vi "Test Publisher.vi"() -> ()   [LabVIEW 2021]
uses:
  CIFChannels/Typedef/Direction.ctl
  CIF_NIChn_FIFO_DAQ.lvclass
  ChannelCommon/typedef/TimeStamps.ctl
  ChannelCommon/typedef/Datatype Waveform.ctl
  <vilib>/CIF Foundation/CIF Utilities/DataTypes/Flatten U64.vi
  CIFChannels/CIFChannels.lvclass
  ChannelCommon/ChannelCommon.lvlib
panel:
  in  "stop":bool
  out "timed out?":bool
  out "error out":errorcluster
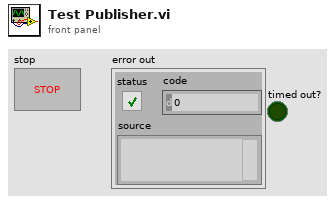
[diagram p1: front panel]
types:
  T1 = typedef "CIFChannels.lvclass/Direction.ctl" = enum16{"Publisher", "Subscriber"}
  T2 = typedef "ChannelCommon.lvlib/Datatype Waveform.ctl" = cluster{"measurement":dbl[], "dT":dbl, "Timestamp":i64, "Read Lock":bool}
  T3 = typedef "ChannelCommon.lvlib/TimeStamps.ctl" = cluster{"ClockID":u8, "T0":i64, "T_Out":i64}
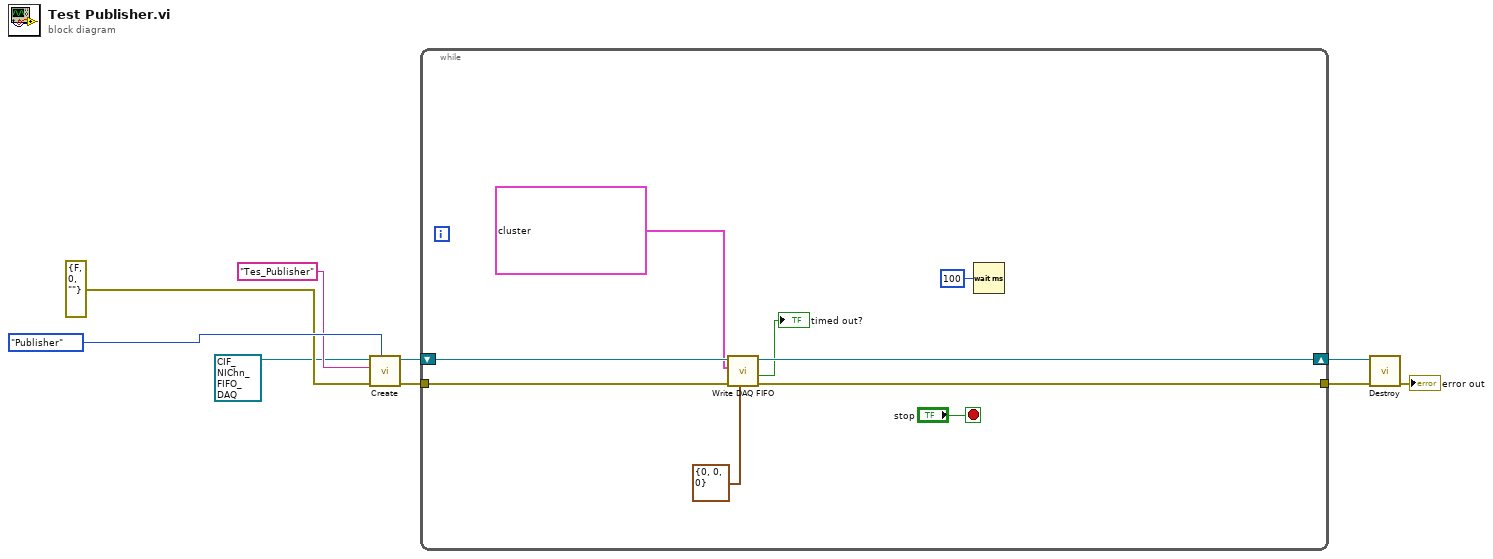
[diagram p0: block diagram]
diagram:
  n1 = call-dynamic "Create.vi"("Direction"=Direction."Publisher", "error in (no error)"=errorcluster {"status"=FALSE, "code"=0, "source"=""} ("error out"), "Name"="Tes_Publisher", "CIFFIFO in"=refnum<class "CIF_NIChn_FIFO_DAQ.lvclass"> refnum ("CIF_NIChn_FIFO_DAQ.lvclass")) -> ("error out"=w5:errorcluster, "CIFFIFO out"=w6:refnum<class "CIF_NIChn_FIFO_DAQ.lvclass">)  [unwired: 6 in]
  n2 = while {
    shift-right: [w15] -> w4
    shift-left: w6 -> [w17]
    tunnel: w5 -> [w16]
    tunnel: [w14] -> w3
    stop <- "stop" stop-if-true
    n3 = call-dynamic "Write DAQ FIFO.vi"("FIFO Timestamps"=T3 {"ClockID"=0, "T0"=0, "T_Out"=0}, "error in (no error)"=w16, "Data In"=T2[] [{"measurement"=array[986 elements], "dT"=43.0, "Timestamp"=2, "Read Lock"=FALSE}, {"measurement"=array[1001 elements], "dT"=34.0, "Timestamp"=1, "Read Lock"=FALSE}, {"measurement"=[], "dT"=0.0, "Timestamp"=0, "Read Lock"=FALSE}, {"measurement"=[], "dT"=0.0, "Timestamp"=0, "Read Lock"=FALSE}, {"measurement"=[], "dT"=0.0, "Timestamp"=0, "Read Lock"=FALSE}, {"measurement"=[], "dT"=0.0, "Timestamp"=0, "Read Lock"=FALSE}, {"measurement"=[], "dT"=0.0, "Timestamp"=0, "Read Lock"=FALSE}, {"measurement"=[], "dT"=0.0, "Timestamp"=0, "Read Lock"=FALSE}, {"measurement"=array[100001 elements], "dT"=0.0, "Timestamp"=0, "Read Lock"=FALSE}] ("DAQ In"), "CIF_NIChn_FIFO_DAQ in"=w17) -> ("error out"=w14:errorcluster, "timed out?"=→"timed out?":bool, "CIF_NIChn_FIFO_DAQ out"=w15:refnum<class "CIF_NIChn_FIFO_DAQ.lvclass">)  [unwired: 4 in, 1 out]
    n4 = Wait (ms)(milliseconds to wait=u32 100) -> ()  [unwired: 1 out]
  }
  n5 = call-dynamic "Destroy.vi"("error in (no error)"=w3, "CIFFIFO in"=w4) -> ("error out"=→"error out":errorcluster)  [unwired: 8 in, 1 out]
